vi "Set Led(SubVI) Dani.vi"(8 "error in (no error)":errorcluster, 10 "Led Option":T1) -> (0 "error out":errorcluster)   [LabVIEW 2015]
uses:
  Controls/Led Control.ctl
  TypeDefs Host/Handle Enum.ctl
  libkinect_wrapper.dll
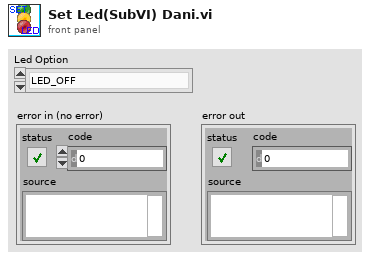
[diagram p1: front panel]
types:
  T1 = typedef "Led Control.ctl" = enum32{"LED_OFF", "LED_GREEN", "LED_RED", "LED_YELLOW", "LED_BLINK_GREEN", "LED_BLINK_GREEN2", "LED_BLINK_RED_YELLOW"}
  T2 = typedef "Handle Enum.ctl" = enum16{"Set Handles", "Get Handles"}
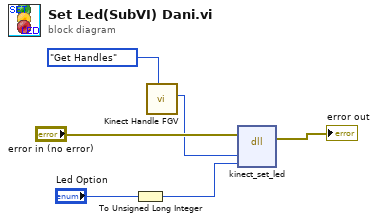
[diagram p0: block diagram]
diagram:
  n1 = To Unsigned Long Integer(number="Led Option") -> (unsigned 32bit integer=w3:u32)
  n2 = call "Kinect Handle FGV.vi"("Handle Command"=Handle_Enum."Get Handles") -> ("Context Handle Out"=w1:i64)  [unwired: 9 in, 1 out]
  n3 = dll-call lib="libkinect_wrapper.*" fn="kinect_set_led"(error in="error in (no error)", "handle"=w1, "option"=w3) -> (error out=→"error out":errorcluster)  [unwired: 5 in, 1 out]
